vi "Send MirrorMoved.vi"(7 "Message Priority (Normal)":T2=enum."Normal", 8 "error in (no error)":errorcluster, 9 "Front/Side":bool, 10 "Mirror":T1, 11 "Message Enqueuer":refnum<class "Message Enqueuer.lvclass">) -> (0 "error out":errorcluster, 3 "Message Enqueuer out":refnum<class "Message Enqueuer.lvclass">)   [LabVIEW 2023, in "MirrorMoved Msg.lvclass"]
doc: "This VI sends the message to an actor."
uses:
  MirrorMoved Msg.lvclass
  MirrorMoved Msg.lvclass/MirrorMoved Msg.ctl
  <vilib>/ActorFramework/Message Enqueuer/Message Enqueuer.lvclass
  Applications/National Instruments/LabVIEW 2023 64-bit/vi.lib/ActorFramework/Message/Message.lvclass
  Users/alexandrosspiliotis/Documents/LV_DAQ_Project/Interfaces/AbstractInstrumentClasses/Spectrometers_LV/SpectrometerComm Messages/MirrorMoved Msg/MirrorMoved Msg.lvclass
  <vilib>/ActorFramework/Message Enqueuer/Message Priority.ctl
  UIs/SpectroscopyUI/SpectroscopyUI/SpectroMirrorCtrl.ctl
  UIs/SpectroscopyUI/SpectroscopyUI.lvlib
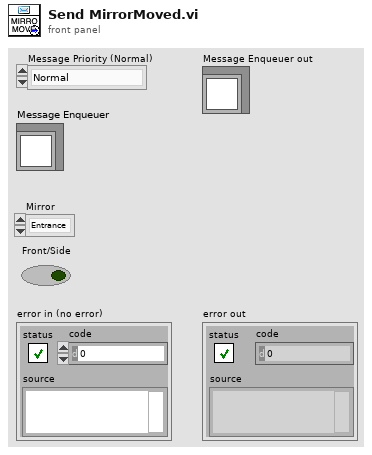
[diagram p1: front panel]
types:
  T1 = typedef "SpectroscopyUI.lvlib/SpectroMirrorCtrl.ctl" = enum16{"Entrance", "Exit"}
  T2 = typedef "Actor Framework.lvlib/Message Enqueuer.lvclass/Message Priority.ctl" = enum16{"Low", "Normal", "High"}
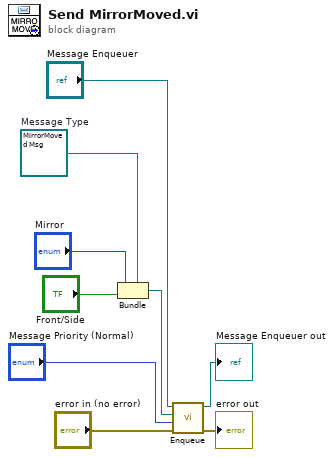
[diagram p0: block diagram]
diagram:
  w6 = refnum<class "MirrorMoved Msg.lvclass"> refnum  # Message Type
  n1 = Bundle(cluster=w6, "Mirror", "Front/Side") -> (w5:refnum<class "MirrorMoved Msg.lvclass">)
  n2 = call <vilib>:"Enqueue.vi"("error in (no error)"="error in (no error)", "Message Priority (Normal)"="Message Priority (Normal)", "Message"=w5, "Message Enqueuer in"="Message Enqueuer") -> ("error out"=→"error out":errorcluster, "Message Enqueuer out"=→"Message Enqueuer out":refnum<class "Message Enqueuer.lvclass">)  [unwired: 6 in]
